vi "Generate Tone.vi"(9 "Duration (1 second)":dbl=1.0, 10 "Frequency (500 Hz)":dbl=500.0) -> (3 "Single Tone out":refnum<class "Single Tone.lvclass">)   [LabVIEW 2017, in "Single Tone.lvclass"]
doc: "This method sets the parameters that will be used to create a waveform for Single Tone."
uses:
  Single Tone.lvclass
  Single Tone.lvclass/Single Tone.ctl
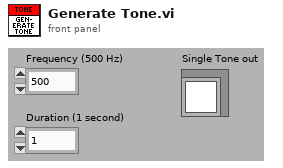
[diagram p1: front panel]
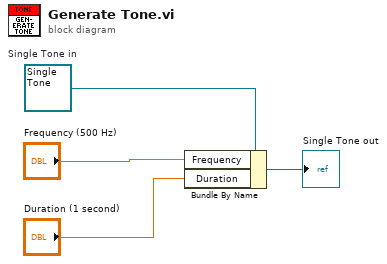
[diagram p0: block diagram]
diagram:
  w4 = refnum<class "Single Tone.lvclass"> refnum  # Single Tone in
  n1 = Bundle By Name(cluster=w4, "Frequency"="Frequency (500 Hz)", "Duration"="Duration (1 second)") -> (→"Single Tone out":refnum<class "Single Tone.lvclass">)
